vi "Get SequenceFile.vi"(8 "error in (no error)":errorcluster, 11 "SequenceViewPanel in":refnum<class "SequenceViewPanel.lvclass">) -> (0 "error out":errorcluster, 2 "SequenceFile":refnum<class "SequenceFile.lvclass">, 3 "SequenceViewPanel out":refnum<class "SequenceViewPanel.lvclass">)   [LabVIEW 2020, in "TSnax UI.lvlib" / "SequenceViewPanel.lvclass"]
uses:
  SequenceViewPanel.lvclass
  SequenceViewPanel.lvclass/SequenceViewPanel.ctl
  TSnax/SequenceFile/SequenceFile.lvclass
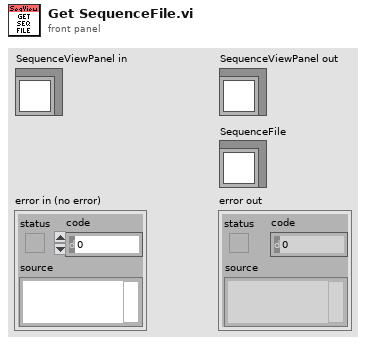
[diagram p1: front panel]
types:
  T1 = typedef "TSnax UI.lvlib/SequenceViewPanel.lvclass/Ref Data.ctl" = cluster{"Insert Index":i32, "SequenceFile":refnum<class "SequenceFile.lvclass">}
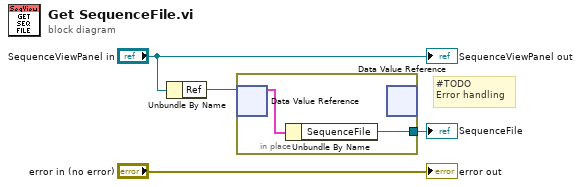
[diagram p0: block diagram]
diagram:
  # "#TODO\nError handling"
  n1 = Unbundle By Name("SequenceViewPanel in") -> ("Ref"=w3:refnum<data-value>)
  n2 = in-place {
    in-place-border: [w5] -> w1
    n3 = in-place-dvr #1(w3) -> (w6:T1)  [unwired: 1 out]
    n4 = Unbundle By Name(w6) -> ("SequenceFile"=w5:refnum<class "SequenceFile.lvclass">)
    n5 = in-place-dvr #1() -> ()  [unwired: 1 in, 2 out]
  }
  "SequenceFile" <- w1
  "error out" <- "error in (no error)"
  "SequenceViewPanel out" <- "SequenceViewPanel in"
